vi "Log TDMS_Local_1.vi"() -> ()   [LabVIEW 2019]
panel:
  in  "Stop":bool
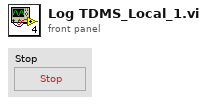
[diagram p1: front panel]
types:
  T1 = enum16{"open", "open or create", "create or replace", "create", "open (read-only)"}
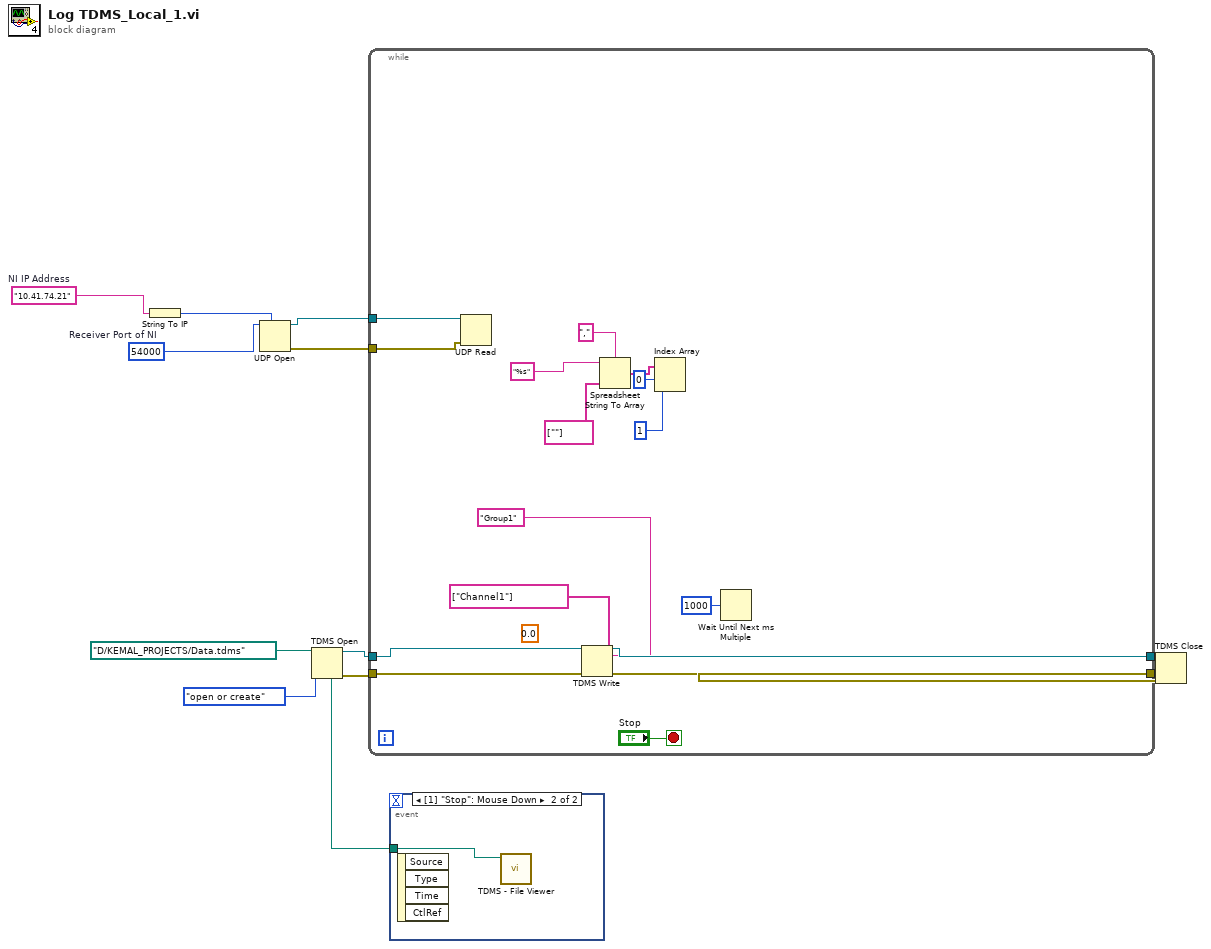
[diagram p0: block diagram]
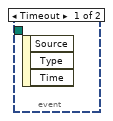
[diagram p2: hidden frame]
diagram:
  w3 = "10.41.74.21"  # NI IP Address
  w5 = u16 54000  # Receiver Port of NI
  w6 = path "D:/KEMAL_PROJECTS/Data.tdms" ("file path")
  n1 = String To IP(1:w3) -> (0:w4:u32)
  n2 = UDP Open(7:w4, 11:w5) -> (port=w2:refnum<k16>, 0:w1:errorcluster)  [unwired: 3 in, 1 out]
  n3 = TDMS Open(10:T1."open or create" ("operation (0:open)"), 11:w6) -> (0:w10:errorcluster, 3:w11:refnum<k34>)  [unwired: 5 in]
  n4 = while {
    tunnel: w11 -> [w27]
    tunnel: [w25] -> w9
    tunnel: w10 -> [w26]
    tunnel: [w24] -> w8
    tunnel: w2 -> [w19]
    tunnel: w1 -> [w18]
    stop <- "Stop" stop-if-true
    (unwired) 0.0
    n5 = UDP Read(connection ID=w19, 8:w18) -> ()  [unwired: 2 in, 5 out]
    n6 = TDMS Write(0:w27, 5:"Group1" ("group name in (Untitled)"), 7:string[] ["Channel1"] ("channel name(s) in (Untitled)"), 11:w26) -> (4:w25:refnum<k34>, 15:w24:errorcluster)  [unwired: 2 in, 2 out]
    n7 = Spreadsheet String To Array(delimiter (Tab)=",", format string="%s", array type (2D Dbl)=string[] [""]) -> (array=w16:string[])  [unwired: 1 in]
    n8 = Index Array(array=w16, index #1=0 ("index"), index #2=1 ("index")) -> ()  [unwired: 2 out]
    n9 = Wait Until Next ms Multiple(millisecond multiple=u32 1000) -> ()  [unwired: 1 out]
  }
  n10 = event shown="[1] \"Stop\": Mouse Down" {
    selector: _ -> [_ _]
    dyn-events: _ -> [_ _]
    timeout: _ -> [_ _]
    tunnel: w6 -> [_ w28]
    event Timeout {
      n11 = event-data() -> ()  [unwired: 1 in, 3 out]
    }
    event "Stop": Mouse Down {
      n12 = event-data() -> ()  [unwired: 1 in, 4 out]
      n13 = call <vilib>:"TDMS - File Viewer.vi"("file path"=w28) -> ()  [unwired: 5 in, 2 out]
    }
  }
  n14 = TDMS Close(8:w8, 11:w9) -> ()  [unwired: 2 out]
